vi "readLogSettingsApplied.vi"(8 "error in (no error)":errorcluster, 10 "Parser":refnum<class "U8ArrayParserAutoIndexing.lvclass">, 11 "M1M3SAL in":refnum<class "M1M3SAL.lvclass">) -> (0 "error out":errorcluster, 2 "EventSettingsApplied":variant, 3 "M1M3SAL out":refnum<class "M1M3SAL.lvclass">)   [LabVIEW 2016, in "M1M3SupportCommunicator.lvlib" / "M1M3SAL.lvclass"]
uses:
  M1M3SAL.lvclass
  Common_RT_Utilities/U8ArrayParserAutoIndexing/U8ArrayParserAutoIndexing.lvclass
  DataTypes/Topics/EventSettingsApplied.ctl
  DataTypes/Topics/Parts/Timestamp.ctl
  DataTypes/Topics/M1M3SupportTopics.lvlib
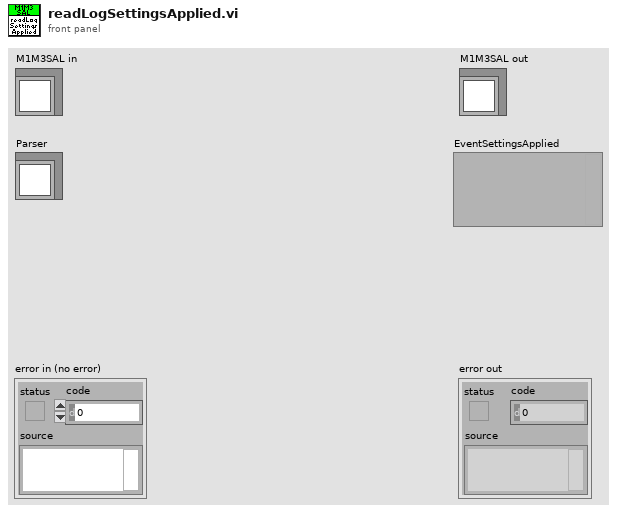
[diagram p1: front panel]
types:
  T1 = typedef "M1M3SupportTopics.lvlib/EventSettingsApplied.ctl" = cluster{"Timestamp":T2, "Settings":string}
  T2 = typedef "M1M3SupportTopics.lvlib/Timestamp.ctl" = dbl
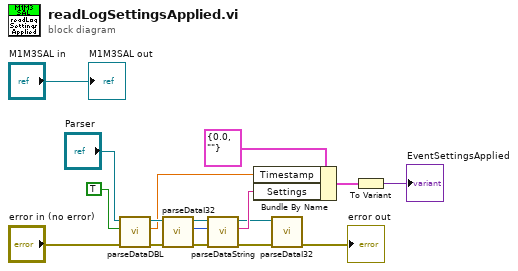
[diagram p0: block diagram]
diagram:
  n1 = call "parseDataDBL.vi"("error in (no error)"="error in (no error)", "OverrideSwapBytes"=TRUE, "U8ArrayParserAutoIndexing in"="Parser") -> ("error out"=w10:errorcluster, "Data"=w8:dbl, "U8ArrayParserAutoIndexing out"=w9:refnum<class "U8ArrayParserAutoIndexing.lvclass">)  [unwired: 6 in]
  n2 = call "parseDataI32.vi"("error in (no error)"=w10, "U8ArrayParserAutoIndexing in"=w9) -> ("error out"=w1:errorcluster, "Data"=w6:i32, "U8ArrayParserAutoIndexing out"=w5:refnum<class "U8ArrayParserAutoIndexing.lvclass">)  [unwired: 7 in]
  n3 = call "parseDataString.vi"("error in (no error)"=w1, "Length"=w6, "U8ArrayParserAutoIndexing in"=w5) -> ("error out"=w2:errorcluster, "Data"=w4:string, "U8ArrayParserAutoIndexing out"=w3:refnum<class "U8ArrayParserAutoIndexing.lvclass">)  [unwired: 6 in]
  n4 = Bundle By Name(cluster=T1 {"Timestamp"=0.0, "Settings"=""} ("EventSettingsApplied"), "Timestamp"=w8, "Settings"=w4) -> (w16:T1)
  n5 = call "parseDataI32.vi"("error in (no error)"=w2, "U8ArrayParserAutoIndexing in"=w3) -> ("error out"=→"error out":errorcluster)  [unwired: 7 in, 2 out]
  n6 = To Variant(anything=w16) -> (Variant=→"EventSettingsApplied":variant)
  "M1M3SAL out" <- "M1M3SAL in"
